vi "test-trajectory-generator-get.vi"(11 "traj_config":T4={"MaxVelocity"=0.0, "Max Acceleration"=0.0, "StartVelocity"=0.0, "End Velocity"=0.0, "Reversed"=FALSE, "DiffDrKineConstntDefined"=FALSE, "CentAcellConstntDefined"=FALSE, "DiffDrVoltConstntDefined"=FALSE, "DIFF_DRIVE_KINE_CONSTRAINT"={"Max Speed (M/S)"=0.0, "DIFF_DRIVE_KINEMATICS"={"TrackWidth_Meters"=0.0}, "Max Accel (M/S2)"=99999.0}, "CENTRIPETAL_ACCEL_CONSTRAINT"={"Max Cent Accel"=0.0}, "SwerveDrKineConstntDefined"=FALSE, "SWERVE_DRIVE_KINE_CONSTRAINT"={"Max Speed (M/S)"=0.0, "SwerveKinematics"={"NumModules"=0, "InverseKinematics"=[], "ForwardKinematics"=[], "Modules"=[], "PrevCoR"={"X"=0.0, "Y"=0.0}}}, "DIFF_DRIVE_VOLTAGE_CONSTRAINT"={"Max Voltage"=0.0, "DIFF_DRIVE_KINEMATICS"={"TrackWidth_Meters"=0.0}, "SIMPLE_MOTOR_FF"={"Ks"=0.0, "Kv"=0.0, "Ka"=0.0}}, "MECANUM_DRIVE_KINE_CONSTRAINT"={"Max Speed (M/S)"=0.0, "MECA_DRIVE_KINEMATICS"={"FrontLeft"={"X"=0.0, "Y"=0.0}, "FrontRight"={"X"=0.0, "Y"=0.0}, "RearLeft"={"X"=0.0, "Y"=0.0}, "RearRight"={"X"=0.0, "Y"=0.0}, "InverseKinematics"=[[0.0, 1.0, -1.0, 0.0], [0.0, 1.0, 1.0, 0.0], [0.0, 1.0, 1.0, 0.0], [0.0, 1.0, -1.0, 0.0]], "ForwardKinematics"=[[0.0, 1.0, -1.0, 0.0], [0.0, 1.0, 1.0, 0.0], [0.0, 1.0, 1.0, 0.0], [0.0, 1.0, -1.0, 0.0]], "PrevCoR"={"X"=0.0, "Y"=0.0}}}, "MecanumDrKineConstntDefined"=FALSE} {"MECANUM_DRIVE_KINE_CONSTRAINT"."MECA_DRIVE_KINEMATICS"."PrevCoR"."Y" format="%14.3f"; "MECANUM_DRIVE_KINE_CONSTRAINT"."MECA_DRIVE_KINEMATICS"."PrevCoR"."X" format="%14.3f"; "MECANUM_DRIVE_KINE_CONSTRAINT"."MECA_DRIVE_KINEMATICS"."RearRight"."Y" format="%14.3f"; "MECANUM_DRIVE_KINE_CONSTRAINT"."MECA_DRIVE_KINEMATICS"."RearRight"."X" format="%14.3f"; "MECANUM_DRIVE_KINE_CONSTRAINT"."MECA_DRIVE_KINEMATICS"."RearLeft"."Y" format="%14.3f"; "MECANUM_DRIVE_KINE_CONSTRAINT"."MECA_DRIVE_KINEMATICS"."RearLeft"."X" format="%14.3f"; "MECANUM_DRIVE_KINE_CONSTRAINT"."MECA_DRIVE_KINEMATICS"."FrontRight"."Y" format="%14.3f"; "MECANUM_DRIVE_KINE_CONSTRAINT"."MECA_DRIVE_KINEMATICS"."FrontRight"."X" format="%14.3f"; "MECANUM_DRIVE_KINE_CONSTRAINT"."MECA_DRIVE_KINEMATICS"."FrontLeft"."Y" format="%14.3f"; "MECANUM_DRIVE_KINE_CONSTRAINT"."MECA_DRIVE_KINEMATICS"."FrontLeft"."X" format="%14.3f"; "MECANUM_DRIVE_KINE_CONSTRAINT"."Max Speed (M/S)" format="%20.4f"; "DIFF_DRIVE_VOLTAGE_CONSTRAINT"."SIMPLE_MOTOR_FF"."Ka" format="%13.4f"; "DIFF_DRIVE_VOLTAGE_CONSTRAINT"."SIMPLE_MOTOR_FF"."Kv" format="%13.4f"; "DIFF_DRIVE_VOLTAGE_CONSTRAINT"."SIMPLE_MOTOR_FF"."Ks" format="%13.4f"; "DIFF_DRIVE_VOLTAGE_CONSTRAINT"."DIFF_DRIVE_KINEMATICS"."TrackWidth_Meters" format="%20.4f"; "DIFF_DRIVE_VOLTAGE_CONSTRAINT"."Max Voltage" format="%20.4f"; "SWERVE_DRIVE_KINE_CONSTRAINT"."SwerveKinematics"."PrevCoR"."Y" format="%14.3f"; "SWERVE_DRIVE_KINE_CONSTRAINT"."SwerveKinematics"."PrevCoR"."X" format="%14.3f"; "SWERVE_DRIVE_KINE_CONSTRAINT"."SwerveKinematics"."Modules"."Y" format="%14.3f"; "SWERVE_DRIVE_KINE_CONSTRAINT"."SwerveKinematics"."Modules"."X" format="%14.3f"; "SWERVE_DRIVE_KINE_CONSTRAINT"."Max Speed (M/S)" format="%20.4f"; "CENTRIPETAL_ACCEL_CONSTRAINT"."Max Cent Accel" format="%20.4f"; "DIFF_DRIVE_KINE_CONSTRAINT"."Max Accel (M/S2)" format="%20.4f"; "DIFF_DRIVE_KINE_CONSTRAINT"."DIFF_DRIVE_KINEMATICS"."TrackWidth_Meters" format="%20.4f"; "DIFF_DRIVE_KINE_CONSTRAINT"."Max Speed (M/S)" format="%20.4f"; "End Velocity" format="%20.4f"; "StartVelocity" format="%20.4f"; "Max Acceleration" format="%20.4f"; "MaxVelocity" format="%20.4f"}) -> (0 "error out":errorcluster, 3 "TRAJECTORY":T15 {"States"."POSE"."ROTATION"."SIN" format="%13.4f"; "States"."POSE"."ROTATION"."COS" format="%13.4f"; "States"."POSE"."ROTATION"."VALUE" format="%13.4f"; "States"."POSE"."TRANSLATION"."Y" format="%14.3f"; "States"."POSE"."TRANSLATION"."X" format="%14.3f"; "TotalTImeSecs" format="%20.3f"}, 4 "Waypoints":T1[](array[typedef]) {"ROTATION"."SIN" format="%13.4f"; "ROTATION"."COS" format="%13.4f"; "ROTATION"."VALUE" format="%13.4f"; "TRANSLATION"."Y" format="%14.3f"; "TRANSLATION"."X" format="%14.3f"})   [LabVIEW 2019]
uses:
  <vilib>/Rock Robotics/WPI/ThirdParty/JAS_Junk/TrajLib/TRAJECTORY.ctl
  <vilib>/Rock Robotics/WPI/ThirdParty/JAS_Junk/TrajLib/TRAJ_STATE.ctl
  <vilib>/Rock Robotics/WPI/ThirdParty/JAS_Junk/TrajLib/POSE2D.ctl
  <vilib>/Rock Robotics/WPI/ThirdParty/JAS_Junk/TrajLib/TRANSLATION2D.ctl
  <vilib>/Rock Robotics/WPI/ThirdParty/JAS_Junk/TrajLib/ROTATION2D.ctl
  <vilib>/Rock Robotics/WPI/ThirdParty/JAS_Junk/TrajLib/TRAJ_CONFIG.ctl
  <vilib>/Rock Robotics/WPI/ThirdParty/JAS_Junk/TrajLib/TRAJ_CONSTRAINT_DIIF_DRIVE_KINEMATICS.ctl
  <vilib>/Rock Robotics/WPI/ThirdParty/JAS_Junk/TrajLib/DIFF_DRIVE_KINEMATICS.ctl
  <vilib>/Rock Robotics/WPI/ThirdParty/JAS_Junk/TrajLib/TRAJ_CONSTRAINT_CENTRIPETAL_ACCEL.ctl
  <vilib>/Rock Robotics/WPI/ThirdParty/JAS_Junk/TrajLib/TRAJ_CONSTRAINT_SWERVE_DRIVE_KINEMATICS.ctl
  <vilib>/Rock Robotics/WPI/ThirdParty/JAS_Junk/TrajLib/SWERVE_DRIVE_KINEMATICS.ctl
  <vilib>/Analysis/Matrix/Datatypes/RealMatrix.ctl
  <vilib>/Rock Robotics/WPI/ThirdParty/JAS_Junk/TrajLib/TRAJ_CONSTRAINT_DIIF_DRIVE_VOLTAGE.ctl
  <vilib>/Rock Robotics/WPI/ThirdParty/JAS_Junk/TrajLib/SIMPLE_MOTOR_FF.ctl
  <vilib>/Rock Robotics/WPI/ThirdParty/JAS_Junk/TrajLib/TRAJ_CONSTRAINT_MECA_DRIVE_KINEMATICS.ctl
  <vilib>/Rock Robotics/WPI/ThirdParty/JAS_Junk/TrajLib/MECA_DRIVE_KINEMATICS.ctl
  <vilib>/Rock Robotics/WPI/ThirdParty/JAS_Junk/TrajLib/UTIL_WAYPOINT.ctl
  <vilib>/Rock Robotics/WPI/ThirdParty/JAS_Junk/TrajLib/Rotation_CreateAngle.vi
  <vilib>/Rock Robotics/WPI/ThirdParty/JAS_Junk/TrajLib/Pose_TransformBy.vi
  <vilib>/Rock Robotics/WPI/ThirdParty/JAS_Junk/TrajLib/Translation_RotateBy.vi
  <vilib>/Rock Robotics/WPI/ThirdParty/JAS_Junk/TrajLib/Translation_Plus.vi
  <vilib>/Rock Robotics/WPI/ThirdParty/JAS_Junk/TrajLib/Rotation_Plus.vi
  <vilib>/Rock Robotics/WPI/ThirdParty/JAS_Junk/TrajLib/Pose_New_TRRO.vi
  <vilib>/Rock Robotics/WPI/ThirdParty/JAS_Junk/TrajLib/Rotation_RotateBy.vi
  <vilib>/Rock Robotics/WPI/ThirdParty/JAS_Junk/TrajLib/Rotation_CreateXY.vi
  <vilib>/Rock Robotics/WPI/ThirdParty/JAS_Junk/TrajLib/Util_CalcDist.vi
  <vilib>/Rock Robotics/WPI/ThirdParty/JAS_Junk/TrajLib/Trajectory_Library.lvlib
  <vilib>/Analysis/Matrix/NI_Matrix.lvlib
panel:
  # "ARRAY OF OTHER\nCONSTRAINTS \nGOES HERE.."
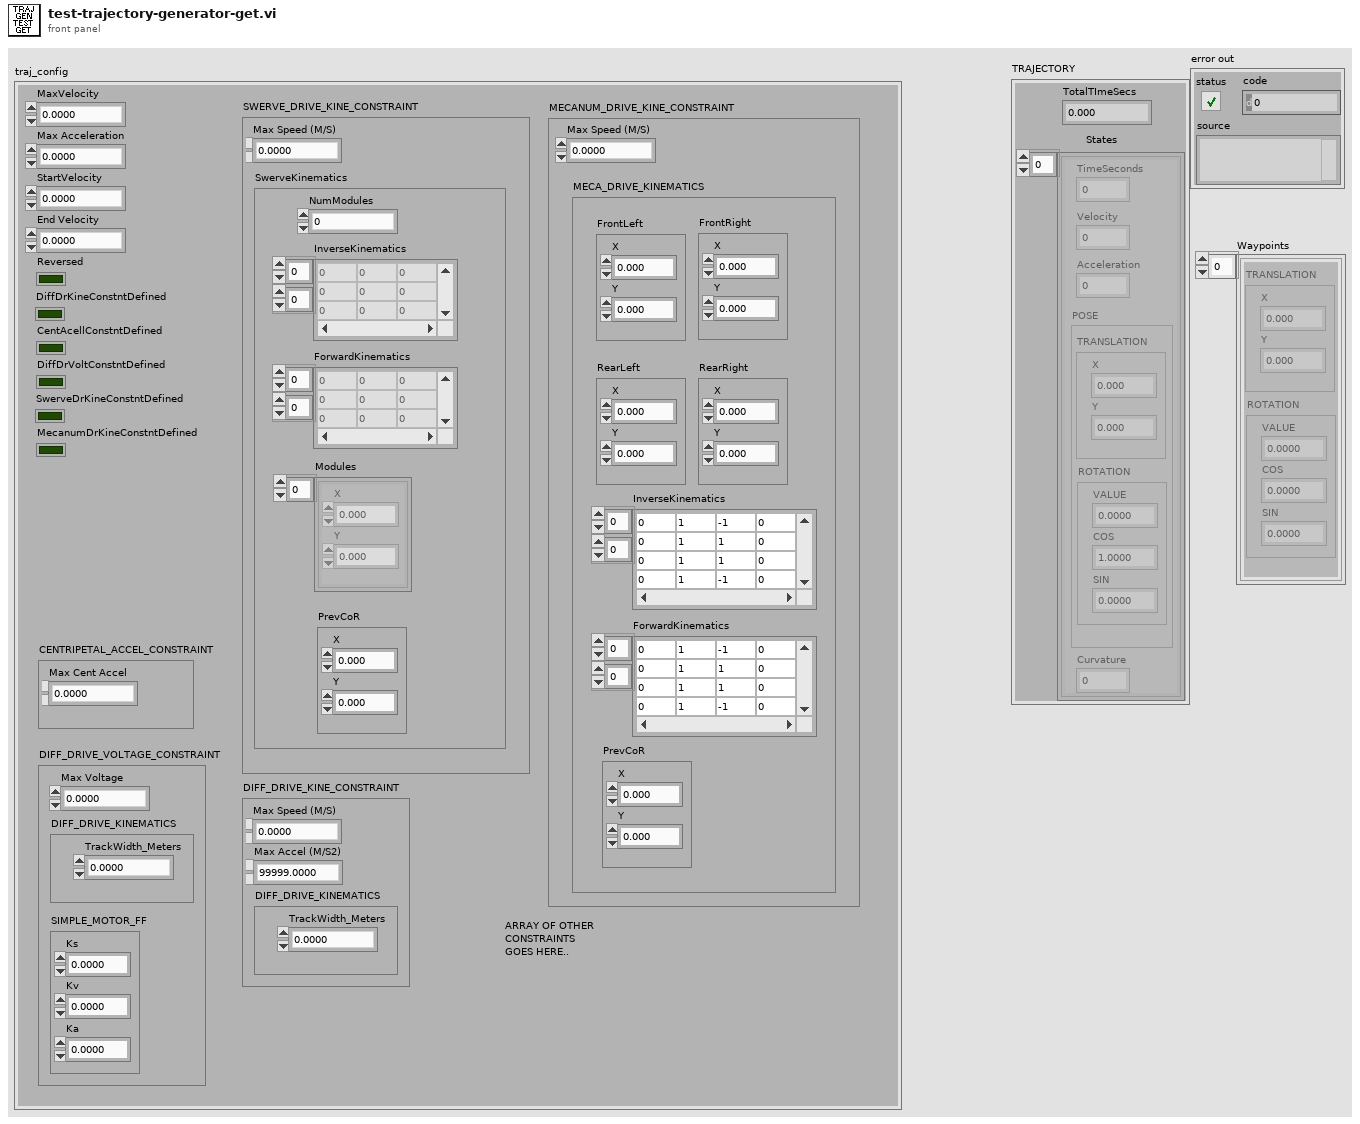
[diagram p1: front panel]
types:
  T1 = typedef "Trajectory_Library.lvlib/POSE2D.ctl" = cluster{"TRANSLATION":T2, "ROTATION":T3}
  T2 = typedef "Trajectory_Library.lvlib/TRANSLATION2D.ctl" = cluster{"X":dbl, "Y":dbl}
  T3 = typedef "Trajectory_Library.lvlib/ROTATION2D.ctl" = cluster{"VALUE":dbl, "COS":dbl, "SIN":dbl}
  T4 = typedef "Trajectory_Library.lvlib/TRAJ_CONFIG.ctl" = cluster{"MaxVelocity":dbl, "Max Acceleration":dbl, "StartVelocity":dbl, "End Velocity":dbl, "Reversed":bool, "DiffDrKineConstntDefined":bool, "CentAcellConstntDefined":bool, "DiffDrVoltConstntDefined":bool, "DIFF_DRIVE_KINE_CONSTRAINT":T5, "CENTRIPETAL_ACCEL_CONSTRAINT":T7, "SwerveDrKineConstntDefined":bool, "SWERVE_DRIVE_KINE_CONSTRAINT":T8, "DIFF_DRIVE_VOLTAGE_CONSTRAINT":T11, "MECANUM_DRIVE_KINE_CONSTRAINT":T13, "MecanumDrKineConstntDefined":bool}
  T5 = typedef "Trajectory_Library.lvlib/TRAJ_CONSTRAINT_DIIF_DRIVE_KINEMATICS.ctl" = cluster{"Max Speed (M/S)":dbl, "DIFF_DRIVE_KINEMATICS":T6, "Max Accel (M/S2)":dbl}
  T6 = typedef "Trajectory_Library.lvlib/DIFF_DRIVE_KINEMATICS.ctl" = cluster{"TrackWidth_Meters":dbl}
  T7 = typedef "Trajectory_Library.lvlib/TRAJ_CONSTRAINT_CENTRIPETAL_ACCEL.ctl" = cluster{"Max Cent Accel":dbl}
  T8 = typedef "Trajectory_Library.lvlib/TRAJ_CONSTRAINT_SWERVE_DRIVE_KINEMATICS.ctl" = cluster{"Max Speed (M/S)":dbl, "SwerveKinematics":T9}
  T9 = typedef "Trajectory_Library.lvlib/SWERVE_DRIVE_KINEMATICS.ctl" = cluster{"NumModules":i32, "InverseKinematics":T10, "ForwardKinematics":T10, "Modules":T2[], "PrevCoR":T2}
  T10 = typedef "NI_Matrix.lvlib/RealMatrix.ctl" = dbl[][]
  T11 = typedef "Trajectory_Library.lvlib/TRAJ_CONSTRAINT_DIIF_DRIVE_VOLTAGE.ctl" = cluster{"Max Voltage":dbl, "DIFF_DRIVE_KINEMATICS":T6, "SIMPLE_MOTOR_FF":T12}
  T12 = typedef "Trajectory_Library.lvlib/SIMPLE_MOTOR_FF.ctl" = cluster{"Ks":dbl, "Kv":dbl, "Ka":dbl}
  T13 = typedef "Trajectory_Library.lvlib/TRAJ_CONSTRAINT_MECA_DRIVE_KINEMATICS.ctl" = cluster{"Max Speed (M/S)":dbl, "MECA_DRIVE_KINEMATICS":T14}
  T14 = typedef "Trajectory_Library.lvlib/MECA_DRIVE_KINEMATICS.ctl" = cluster{"FrontLeft":T2, "FrontRight":T2, "RearLeft":T2, "RearRight":T2, "InverseKinematics":T10, "ForwardKinematics":T10, "PrevCoR":T2}
  T15 = typedef "Trajectory_Library.lvlib/TRAJECTORY.ctl" = cluster{"TotalTImeSecs":dbl, "States":T16[]}
  T16 = typedef "Trajectory_Library.lvlib/TRAJ_STATE.ctl" = cluster{"TimeSeconds":dbl, "Velocity":dbl, "Acceleration":dbl, "POSE":T1, "Curvature":dbl}
  T17 = typedef "Trajectory_Library.lvlib/TRANSFORM2D.ctl" = cluster{"TRANSLATION":T2, "ROTATION":T3}
  T18 = typedef "Trajectory_Library.lvlib/UTIL_WAYPOINT.ctl" = cluster{"X":dbl, "Y":dbl, "ANGLE":dbl}
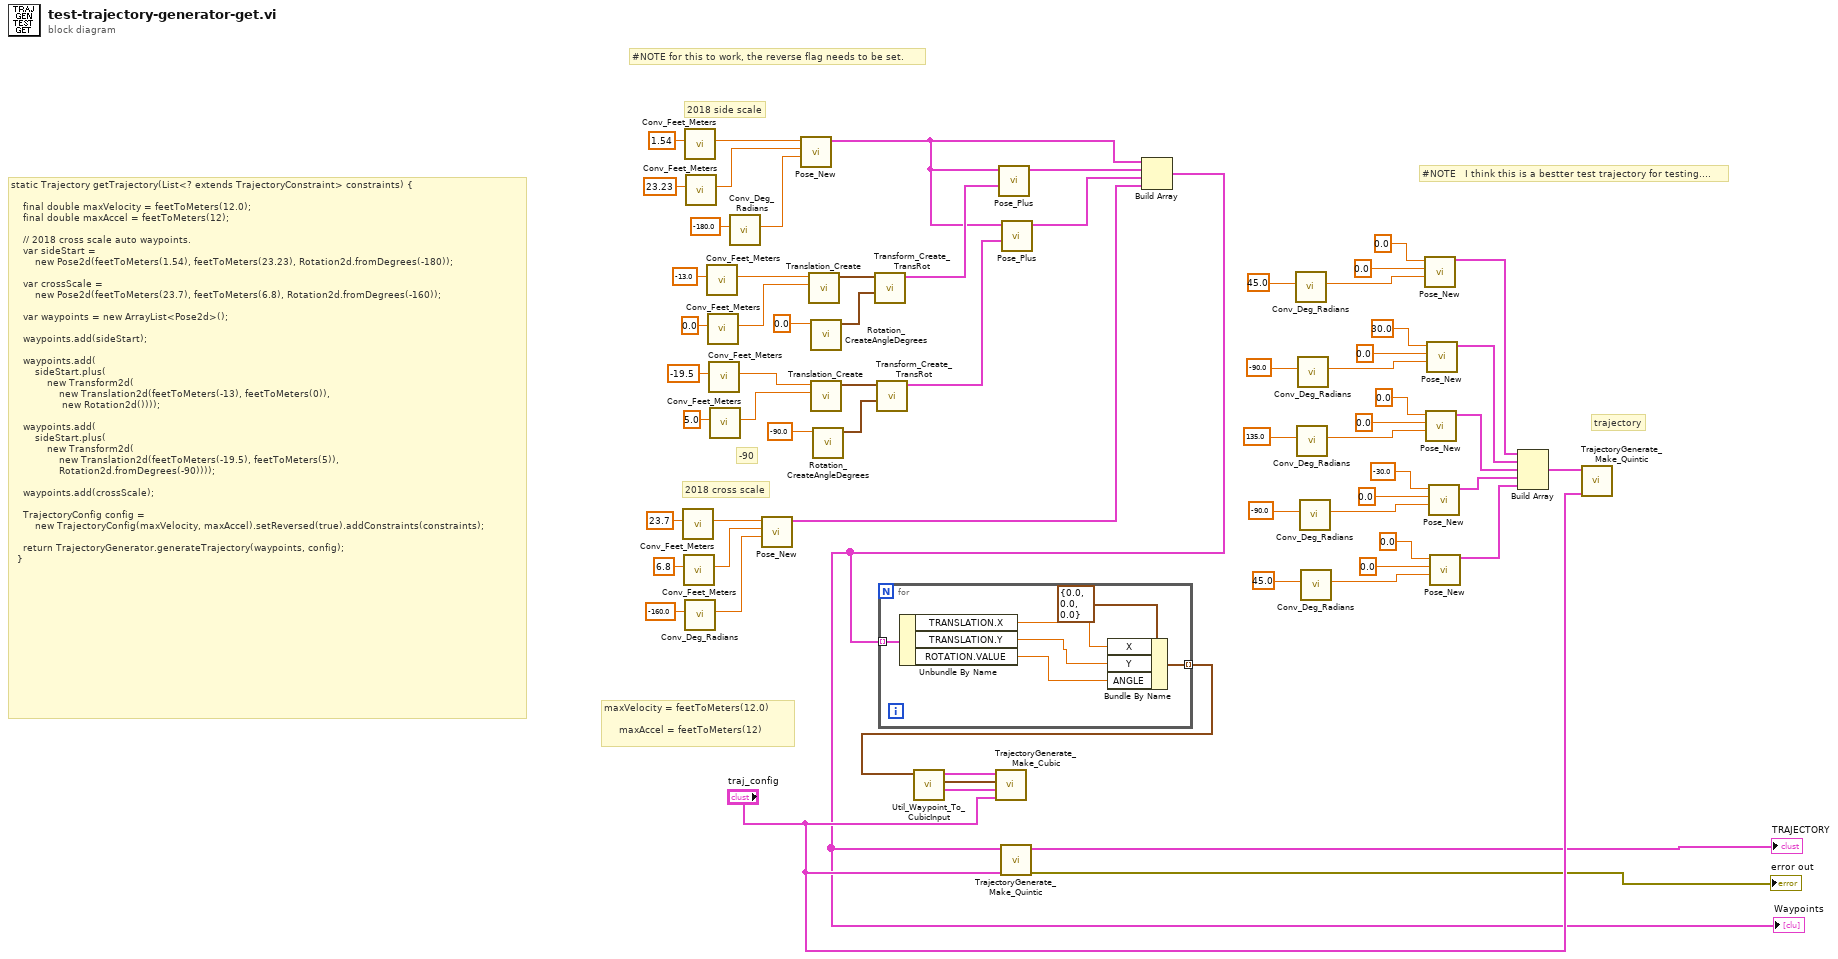
[diagram p0: block diagram]
diagram:
  # "#NOTE for this to work, the reverse flag needs to be set."
  # "-90"
  # "#NOTE   I think this is a bestter test trajectory for testing...."
  # "trajectory"
  # "maxVelocity = feetToMeters(12.0)\n\n     maxAccel = feetToMeters(12)"
  # "2018 cross scale"
  # "2018 side scale"
  # "static Trajectory getTrajectory(List<? extends TrajectoryConstraint> constraints) {\n\n    final double maxVelocity = feetToMeters(12.0);\n    final double maxAccel = feetToMeters(12);\n\n    // 2018 cross scale auto waypoints.\n    var sideStart =\n        new Pose2d(feetToMeters(1.54), feetToMeters(23.23), Rotation2d.fromDegrees(-180));\n\n    var crossScale =\n        new Pose2d(feetToMeters(23.7), feetToMeters(6.8), Rotation2d.fromDegrees(-160));\n\n    var waypoints = new ArrayList<Pose2d>();\n\n    waypoints.add(sideStart);\n\n    waypoints.add(\n        sideStart.plus(\n            new Transform2d(\n                new Translation2d(feetToMeters(-13), feetToMeters(0)), \n                 new Rotation2d())));\n\n    waypoints.add(\n        sideStart.plus(\n            new Transform2d(\n                new Translation2d(feetToMeters(-19.5), feetToMeters(5)),\n                Rotation2d.fromDegrees(-90))));\n\n    waypoints.add(crossScale);\n\n    TrajectoryConfig config =\n        new TrajectoryConfig(maxVelocity, maxAccel).setReversed(true).addConstraints(constraints);\n\n    return TrajectoryGenerator.generateTrajectory(waypoints, config);\n  }"
  n1 = call <vilib>:"Conv_Feet_Meters.vi"("Feet"=23.7) -> ("Meters"=w60:dbl)  [unwired: 10 in]
  n2 = call <vilib>:"Conv_Feet_Meters.vi"("Feet"=6.8) -> ("Meters"=w59:dbl)  [unwired: 10 in]
  n3 = call <vilib>:"Conv_Feet_Meters.vi"("Feet"=1.54) -> ("Meters"=w66:dbl)  [unwired: 10 in]
  n4 = call <vilib>:"Conv_Deg_Radians.vi"("Degress"=-160.0) -> ("Radians"=w58:dbl)  [unwired: 10 in]
  n5 = call <vilib>:"Conv_Feet_Meters.vi"("Feet"=23.23) -> ("Meters"=w65:dbl)  [unwired: 10 in]
  n6 = call <vilib>:"Conv_Feet_Meters.vi"("Feet"=-13.0) -> ("Meters"=w38:dbl)  [unwired: 10 in]
  n7 = call <vilib>:"Conv_Feet_Meters.vi"("Feet"=0.0) -> ("Meters"=w37:dbl)  [unwired: 10 in]
  n8 = call <vilib>:"Conv_Feet_Meters.vi"("Feet"=-19.5) -> ("Meters"=w36:dbl)  [unwired: 10 in]
  n9 = call <vilib>:"Conv_Feet_Meters.vi"("Feet"=5.0) -> ("Meters"=w35:dbl)  [unwired: 10 in]
  n10 = call <vilib>:"Conv_Deg_Radians.vi"("Degress"=-180.0) -> ("Radians"=w64:dbl)  [unwired: 10 in]
  n11 = call <vilib>:"Pose_New.vi"("Heading"=w58, "Y"=w59, "X"=w60) -> ("out POSe"=w54:T1)  [unwired: 8 in]
  n12 = call <vilib>:"Pose_New.vi"("Heading"=w64, "Y"=w65, "X"=w66) -> ("out POSe"=w45:T1)  [unwired: 8 in]
  n13 = call <vilib>:"Translation_Create.vi"("Y"=w37, "X"=w38) -> ("TRANSLATION"=w53:T2)  [unwired: 9 in]
  n14 = call <vilib>:"Rotation_CreateAngleDegrees.vi"("Angle_Degrees"=0.0) -> ("ROTATION"=w52:T3)  [unwired: 10 in]
  n15 = call <vilib>:"Translation_Create.vi"("Y"=w35, "X"=w36) -> ("TRANSLATION"=w48:T2)  [unwired: 9 in]
  n16 = call <vilib>:"Rotation_CreateAngleDegrees.vi"("Angle_Degrees"=-90.0) -> ("ROTATION"=w47:T3)  [unwired: 10 in]
  n17 = call <vilib>:"Transform_Create_TransRot.vi"("ROTATION"=w52, "TRANSLATION"=w53) -> ("TRANSFORM"=w50:T17)  [unwired: 9 in]
  n18 = call <vilib>:"Transform_Create_TransRot.vi"("ROTATION"=w47, "TRANSLATION"=w48) -> ("TRANSFORM"=w44:T17)  [unwired: 9 in]
  n19 = call <vilib>:"Pose_Plus.vi"("other TRANSFORM"=w50, "in POSE"=w45) -> ("out POSE"=w49:T1)  [unwired: 9 in]
  n20 = call <vilib>:"Pose_Plus.vi"("other TRANSFORM"=w44, "in POSE"=w45) -> ("out POSE"=w43:T1)  [unwired: 9 in]
  n21 = Build Array(w45, w49, w43, w54) -> (w3:T1[])
  "Waypoints" <- w3
  n22 = for {
    tunnel: w3 -> [w72] mode=indexing
    tunnel: [w67] -> w31 mode=indexing
    n23 = Unbundle By Name(w72) -> ("TRANSLATION.X"=w68:dbl, "TRANSLATION.Y"=w69:dbl, "ROTATION.VALUE"=w70:dbl)
    n24 = Bundle By Name(cluster=T18 {"X"=0.0, "Y"=0.0, "ANGLE"=0.0} ("UTIL_WAYPOINT"), "X"=w68, "Y"=w69, "ANGLE"=w70) -> (w67:T18)
  }
  n25 = call <vilib>:"Util_Waypoint_To_CubicInput.vi"("WayPoints"=w31) -> ("Final POSE"=w32:T1, "Internal Cubic Waypoints"=w33:T2[], "Initial POSE"=w34:T1)  [unwired: 8 in]
  n26 = call <vilib>:"TrajectoryGenerate_Make_Cubic.vi"("traj_config"="traj_config", "Enging POSE"=w32, "Interior WAYPOINTS"=w33, "Starting POSE"=w34) -> ()  [unwired: 6 in, 2 out]
  n27 = call <vilib>:"TrajectoryGenerate_Make_Quintic.vi"("traj_config"="traj_config", "waypointPOSE"=w3) -> ("error out"=→"error out":errorcluster, "TRAJECTORY"=→"TRAJECTORY":T15)  [unwired: 8 in]
  n28 = call <vilib>:"Conv_Deg_Radians.vi"("Degress"=45.0 ("Heading")) -> ("Radians"=w10:dbl)  [unwired: 10 in]
  n29 = call <vilib>:"Conv_Deg_Radians.vi"("Degress"=135.0 ("Heading")) -> ("Radians"=w18:dbl)  [unwired: 10 in]
  n30 = call <vilib>:"Conv_Deg_Radians.vi"("Degress"=-90.0 ("Heading")) -> ("Radians"=w14:dbl)  [unwired: 10 in]
  n31 = call <vilib>:"Conv_Deg_Radians.vi"("Degress"=-90.0 ("Heading")) -> ("Radians"=w22:dbl)  [unwired: 10 in]
  n32 = call <vilib>:"Conv_Deg_Radians.vi"("Degress"=45.0 ("Heading")) -> ("Radians"=w26:dbl)  [unwired: 10 in]
  n33 = call <vilib>:"Pose_New.vi"("Heading"=w10, "Y"=0.0, "X"=0.0) -> ("out POSe"=w9:T1)  [unwired: 8 in]
  n34 = call <vilib>:"Pose_New.vi"("Heading"=w18, "Y"=0.0, "X"=0.0) -> ("out POSe"=w7:T1)  [unwired: 8 in]
  n35 = call <vilib>:"Pose_New.vi"("Heading"=w14, "Y"=0.0, "X"=30.0) -> ("out POSe"=w8:T1)  [unwired: 8 in]
  n36 = call <vilib>:"Pose_New.vi"("Heading"=w22, "Y"=0.0, "X"=-30.0) -> ("out POSe"=w6:T1)  [unwired: 8 in]
  n37 = call <vilib>:"Pose_New.vi"("Heading"=w26, "Y"=0.0, "X"=0.0) -> ("out POSe"=w28:T1)  [unwired: 8 in]
  n38 = Build Array(w9, w8, w7, w6, w28) -> (w4:T1[])
  n39 = call <vilib>:"TrajectoryGenerate_Make_Quintic.vi"("traj_config"="traj_config", "waypointPOSE"=w4) -> ()  [unwired: 8 in, 2 out]
